vi "Arraystr Fill Format_str.vi"(8 "error in (no error)":errorcluster, 9 "Len":u32, 10 "Format_str":string, 11 "Array":string[](array[string])) -> (0 "error out":errorcluster, 3 "Array str":string[](array[string]))   [LabVIEW 2014]
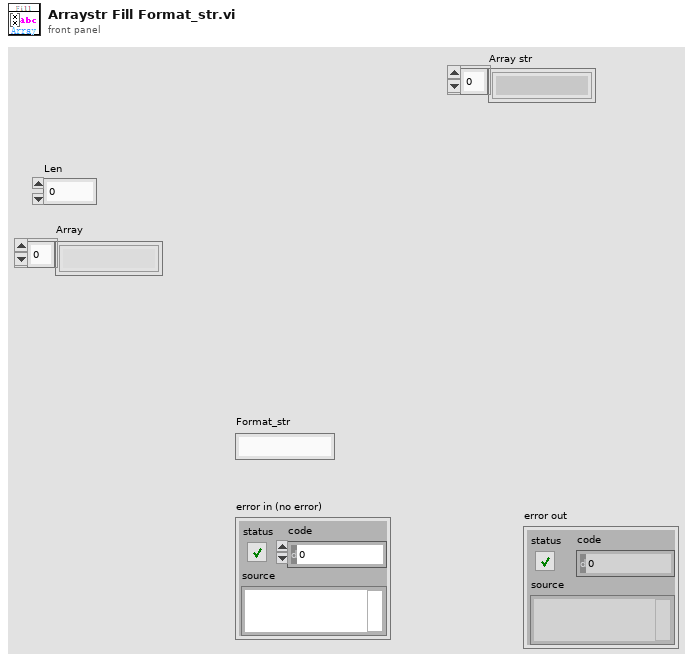
[diagram p1: front panel]
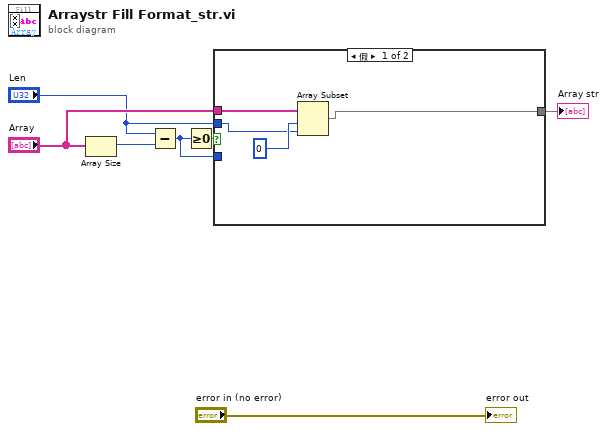
[diagram p0: block diagram]
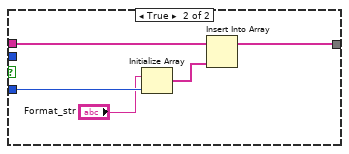
[diagram p2: hidden frame]
diagram:
  n1 = Array Size(array="Array") -> (size(s)=w7:i32)
  n2 = Subtract(x="Len", y=w7) -> (x-y=w4:u32)
  n3 = Greater Or Equal To 0?(x=w4) -> (x >= 0?=w6:bool)
  n4 = case shown="假" w6 {
    tunnel: "Array" -> [w11 w14]
    tunnel: w4 -> [_ w16]
    tunnel: [w8 w12] -> w2
    tunnel: "Len" -> [w9 _]
    frame False {
      n5 = Array Subset(array=w11, index=0, length=w9) -> (w8:string[])
    }
    frame True {
      n6 = Initialize Array("Format_str", w16) -> (w13:string[])
      n7 = Insert Into Array(array=w14, new element=w13) -> (w12:string[])  [unwired: 1 in]
    }
  }
  "Array str" <- w2
  "error out" <- "error in (no error)"
